vi "零点跨度数据组合 (子VI).vi"(6 "数据标识":string="N", 8 "span value":string="0", 9 "standard value":string, 10 "check value":string, 11 "污染物编码":string) -> (3 "组合输出":string)   [LabVIEW 2016, in "数据传输系统-04.lvlib"]
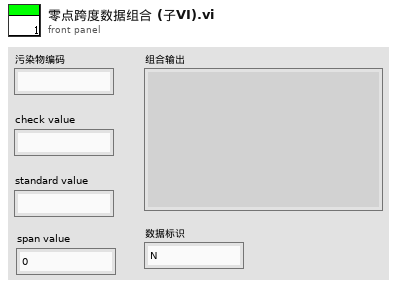
[diagram p1: front panel]
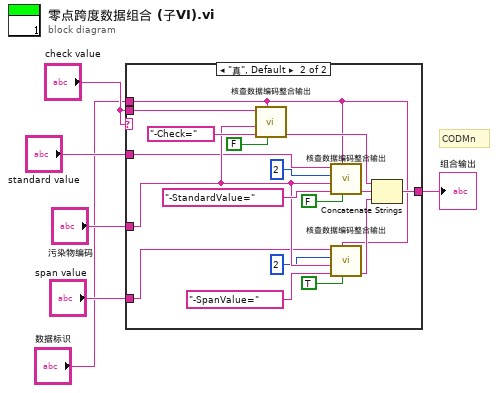
[diagram p0: block diagram]
diagram:
  # "CODMn"
  n1 = case shown="\"真\", Default" "check value" {
    tunnel: "check value" -> [w7 w24]
    tunnel: [w7 w21] -> w3
    tunnel: "standard value" -> [_ w9]
    tunnel: "污染物编码" -> [_ w13]
    tunnel: "span value" -> [_ w10]
    tunnel: "数据标识" -> [_ w8]
    frame "" {
    }
    frame "真", Default {
      n2 = call "核查数据编码整合输出.vi"("字段结束"=FALSE, "数据标识"=w8, "数据类型"="-Check=", "污染物编码"=w13, "数据值"=w24) -> ("编码输出"=w22:string)  [unwired: 6 in]
      n3 = call "核查数据编码整合输出.vi"("字段结束"=FALSE, "数据标识"=w8, "数据类型"="-StandardValue=", "污染物编码"=w13, "数据精度"=2, "数据值"=w9) -> ("编码输出"=w19:string)  [unwired: 5 in]
      n4 = call "核查数据编码整合输出.vi"("字段结束"=TRUE, "数据标识"=w8, "数据类型"="-SpanValue=", "污染物编码"=w13, "数据精度"=2, "数据值"=w10) -> ("编码输出"=w17:string)  [unwired: 5 in]
      n5 = Concatenate Strings(w22, w19, w17) -> (w21:string)
    }
  }
  "组合输出" <- w3
